vi "Write Recipe Data Save Location.vi"(8 "error in (no error)":errorcluster, 10 "Recipe Data Save Location":path, 11 "Recipe State Data in":refnum<class "Recipe State Data.lvclass">) -> (0 "error out":errorcluster, 3 "Recipe State Data out":refnum<class "Recipe State Data.lvclass">)   [LabVIEW 2022 SP3, in "Recipe State Data.lvclass"]
uses:
  Recipe State Data.lvclass
  Recipe State Data.lvclass/Recipe State Data.ctl
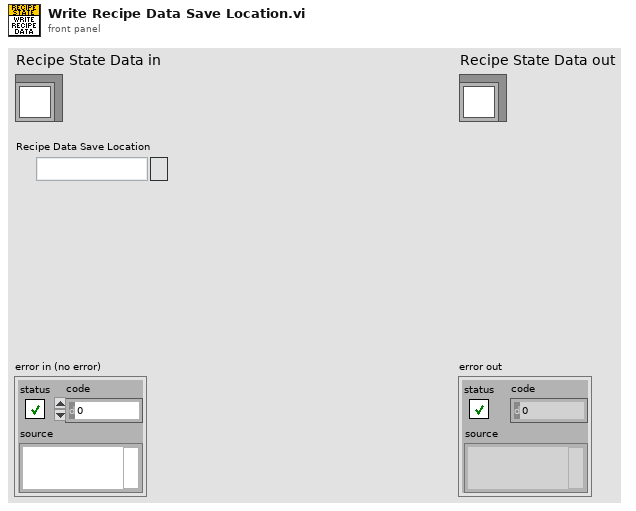
[diagram p1: front panel]
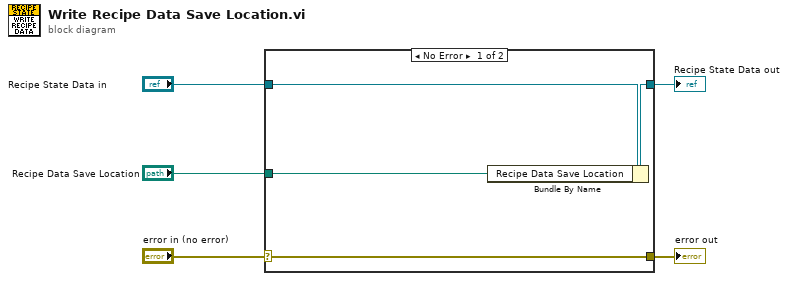
[diagram p0: block diagram]
diagram:
  n1 = case shown="No Error" "error in (no error)" {
    selector: "error in (no error)" -> [w9 w10]
    tunnel: [w9 w10] -> w4
    tunnel: [w7 w11] -> w2
    tunnel: "Recipe State Data in" -> [w8 w11]
    tunnel: "Recipe Data Save Location" -> [w6 _]
    frame No Error {
      n2 = Bundle By Name(cluster=w8, "Recipe Data Save Location"=w6) -> (w7:refnum<class "Recipe State Data.lvclass">)
    }
    frame Error {
    }
  }
  "error out" <- w4
  "Recipe State Data out" <- w2
